vi "Choreo_Choreo_DifferentialLTVCommand.vi"(4 "Pass_Through_Time":dbl=-1.0 format="%33.4f", 5 "TimePastEndSeconds":dbl=3.0, 6 "FlipIfNeeded":bool=TRUE, 8 "Auto":bool=TRUE, 9 "Initialize":bool, 10 "TrajectoryName":string, 11 "Current Position":T3={"TRANSLATION"={"X"=0.0, "Y"=0.0}, "ROTATION"={"VALUE"=0.0, "COS"=1.0, "SIN"=0.0}} {"ROTATION"."SIN" format="%13.4f"; "ROTATION"."COS" format="%13.4f"; "ROTATION"."VALUE" format="%13.4f"; "TRANSLATION"."Y" format="%14.3f"; "TRANSLATION"."X" format="%14.3f"}) -> (0 "Ctrl Info":T1, 1 "Complete":bool, 2 "On Target":bool, 3 "Chassis Speed Dmd":T2 {"vOmega" format="%10.3f"; "vY" format="%10.3f"; "vX" format="%10.3f"})   [LabVIEW 2019, in "ChoreoLib.lvlib"]
doc: "Command to assist in the execution of a Choreo Trajectory. This wraps the ChoreoDifferentialLTVCtrl VI.\n\nInputs:\n - TimePastEndSeconds - double - Number of seconds past the end of the trajectory to continue to control robot position. (Optional. Default: 3.0 )\n - Current Pose - pose2d - Current robot position pose calcualted by either Odometry or Pose Estimation.\n - TrajectoryName - string - Name of trajectory to load from cache. If it isn't in cache, it will try to be loaded from the file system.\n - Initialize - boolean - Set to true for one scan cycle when starting a trajectory. Resets the elapsed time and controllers.\n - Auto - boolean - When TRUE closed loop control is used to control trajectory execution. This is mostly for debugging and robot tuning. (Optional. Default: TRUE )\n - Mirror For Red Alliance - boolean - Whether or not to mirror the path based on alliance (this assumes the path is created for the blue alliance) If TRUE, the alliance color is queried and if RED, the trajectory is flipped for execution.\n - PassThroughTime - double - Continueually counting time (seconds) read from the FGPA on roboRIO or local computer when running on PC. (Optional: Default: Read FGPA time )\n\nOutputs:\n - Choreo Speed Demand - chassis speed - Desired chassis speed (M/S, Rad/Sec)\n - On Target - boolean - TRUE when robot position is within tolerance of trajectory position\n - Complete - boolean - TRUE when trajectory time has elapsed and robot is on target or when trajectory time is \"TimePastEndSeconds\" past trajectory end time regardless of On Target status.\n - Ctrl Info - cluster - Information on control. Mostly for diagnostics."
uses:
  ChoreoLib.lvlib
  <vilib>/Rock Robotics/WPI/ThirdParty/JAS_Junk/TrajLib/TypeDef/POSE2D.ctl
  <vilib>/Rock Robotics/WPI/ThirdParty/JAS_Junk/TrajLib/TypeDef/TRANSLATION2D.ctl
  <vilib>/Rock Robotics/WPI/ThirdParty/JAS_Junk/TrajLib/TypeDef/ROTATION2D.ctl
  <vilib>/Rock Robotics/WPI/ThirdParty/JAS_Junk/TrajLib/TypeDef/CHASSIS_SPEEDS.ctl
  TypeDef/ChoreoTrajectoryDifferential.ctl
  TypeDef/ChoreoDifferentialSample.ctl
  TypeDef/ChoreoEventMarker.ctl
  <vilib>/Rock Robotics/WPI/ThirdParty/JAS_Junk/TrajLib/VI/Util_GetTime_U32.vi
  Choreo_TrajectoryDifferential_Samples.vi
  Choreo_DifferentialSample_GetTimestamp.vi
  <vilib>/Rock Robotics/WPI/ThirdParty/JAS_Junk/TrajLib/VI/Util_GetTime_U64.vi
  <vilib>/Rock Robotics/WPI/DriverStation/WPI_DriverStationGet Alliance Info.vi
  <vilib>/Rock Robotics/WPI/ThirdParty/JAS_Junk/TrajLib/Trajectory_Library.lvlib
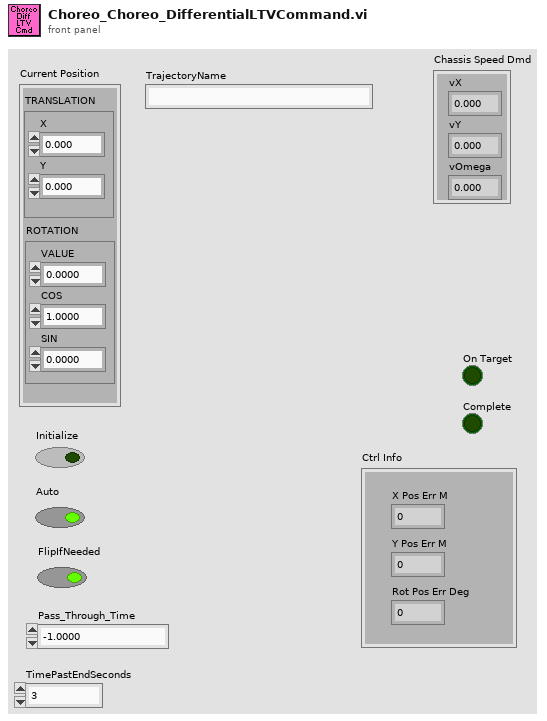
[diagram p1: front panel]
types:
  T1 = cluster{"X Pos Err M":dbl, "Y Pos Err M":dbl, "Rot Pos Err Deg":dbl}
  T2 = typedef "Trajectory_Library.lvlib/CHASSIS_SPEEDS.ctl" = cluster{"vX":dbl, "vY":dbl, "vOmega":dbl}
  T3 = typedef "Trajectory_Library.lvlib/POSE2D.ctl" = cluster{"TRANSLATION":T4, "ROTATION":T5}
  T4 = typedef "Trajectory_Library.lvlib/TRANSLATION2D.ctl" = cluster{"X":dbl, "Y":dbl}
  T5 = typedef "Trajectory_Library.lvlib/ROTATION2D.ctl" = cluster{"VALUE":dbl, "COS":dbl, "SIN":dbl}
  T6 = typedef "ChoreoLib.lvlib/ChoreoTrajectoryDifferential.ctl" = cluster{"name":string, "samples":T7[], "splits":i32[], "events":T8[]}
  T7 = typedef "ChoreoLib.lvlib/ChoreoDifferentialSample.ctl" = cluster{"timestamp":dbl, "x":dbl, "y":dbl, "heading":dbl, "velocityL":dbl, "velocityR":dbl, "angularVelocity":dbl, "accelL":dbl, "accelR":dbl, "accelAngular":dbl, "forceL":dbl, "forceR":dbl}
  T8 = typedef "ChoreoLib.lvlib/ChoreoEventMarker.ctl" = cluster{"TimeStamp":dbl, "Name":string}
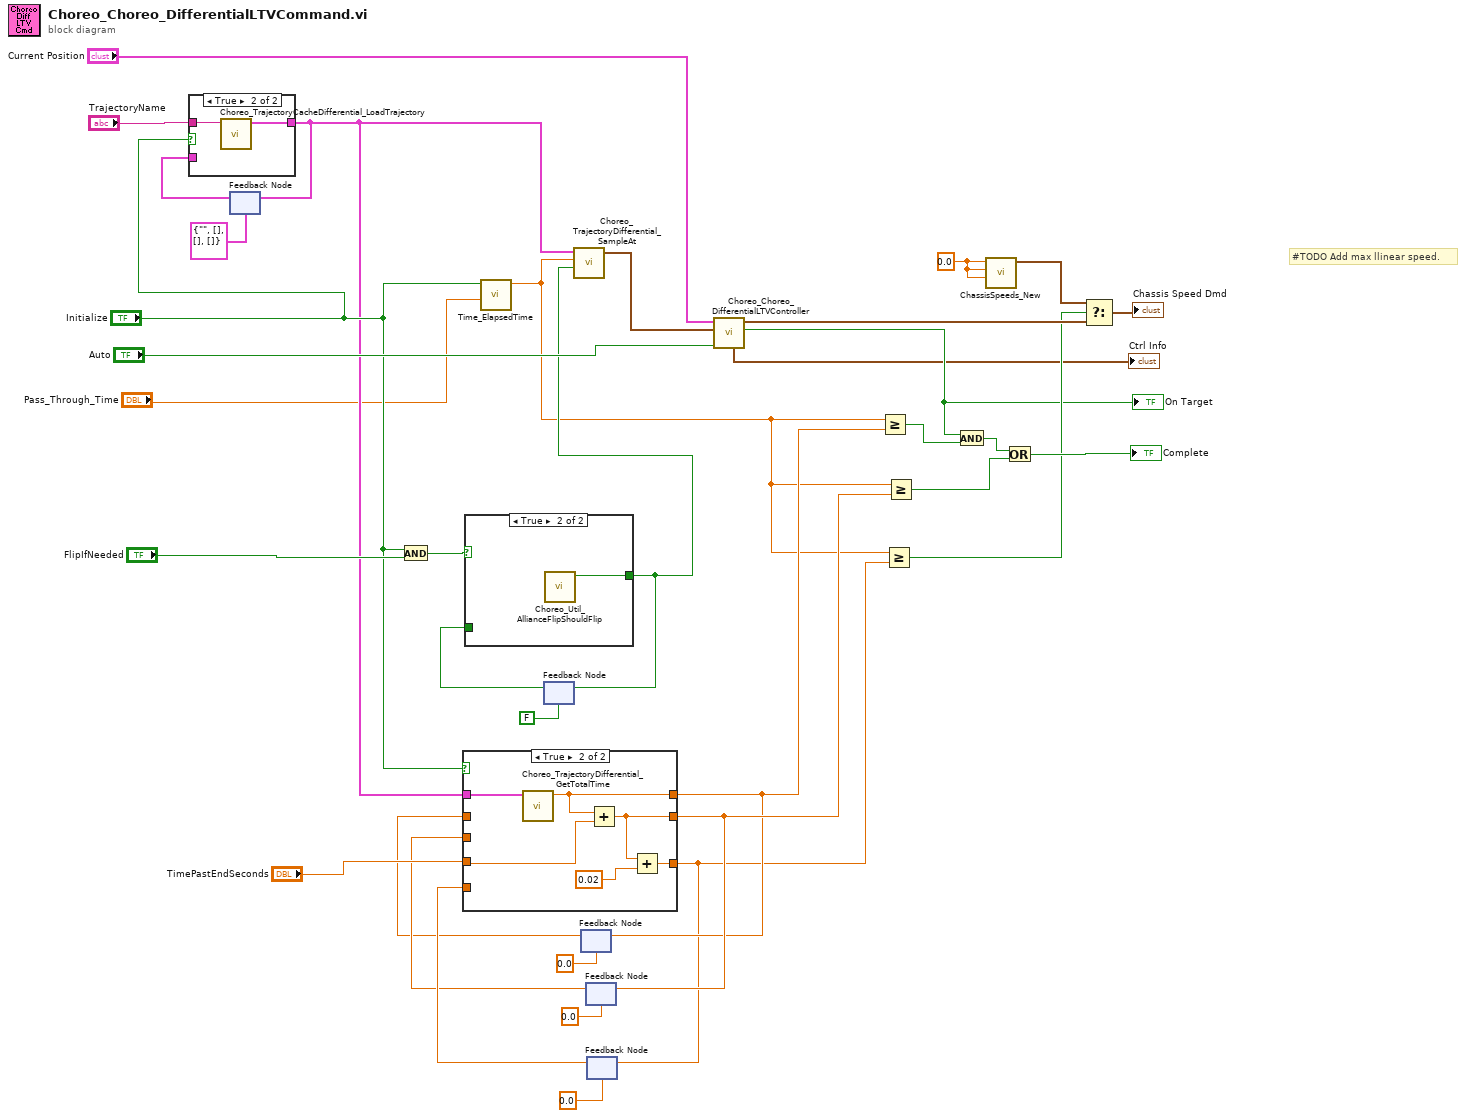
[diagram p0: block diagram]
diagram:
  w10 = 0.0 ("vX")
  # "#TODO Add max llinear speed."
  n1 = feedback #1(T6 {"name"="", "samples"=[], "splits"=[], "events"=[]} ("ChoreoTrajectoryDifferential")) -> (w4:T6)
  n2 = case shown="True" "Initialize" {
    tunnel: [w37 w39] -> w5
    tunnel: "TrajectoryName" -> [_ w38]
    tunnel: w4 -> [w37 _]
    frame False {
    }
    frame True {
      n3 = call "Choreo_TrajectoryCacheDifferential_LoadTrajectory.vi"("TrajectoryName"=w38) -> ("ChoreoTrajectoryDifferential"=w39:T6)  [unwired: 9 in, 1 out]
    }
  }
  n4 = feedback-in #1(w5) -> ()
  n5 = And(x="Initialize", y="FlipIfNeeded") -> (x .and. y?=w32:bool)
  n6 = call <vilib>:"Time_ElapsedTime.vi"("PassthroughTime_SEC"="Pass_Through_Time", "Reset"="Initialize") -> ("Elapsed Time Sec"=w16:dbl)  [unwired: 9 in]
  n7 = feedback #2(FALSE) -> (w30:bool)
  n8 = case shown="True" w32 {
    tunnel: [w40 w41] -> w29
    tunnel: w30 -> [w40 _]
    frame False {
    }
    frame True {
      n9 = call "Choreo_Util_AllianceFlipShouldFlip.vi"() -> ("ShouldFlip"=w41:bool)  [unwired: 11 in]
    }
  }
  n10 = feedback-in #2(w29) -> ()
  n11 = call "Choreo_TrajectoryDifferential_SampleAt.vi"("MirrorForRedAlliance"=w29, "TimeStamp"=w16, "ChoreoTrajectoryDifferential"=w5) -> ("ChoreoDifferentialSample"=w35:T7)  [unwired: 8 in]
  n12 = feedback #3(0.0) -> (w17:dbl)
  n13 = feedback #4(0.0) -> (w24:dbl)
  n14 = feedback #5(0.0) -> (w25:dbl)
  n15 = case shown="True" "Initialize" {
    tunnel: w5 -> [_ w46]
    tunnel: "TimePastEndSeconds" -> [_ w50]
    tunnel: [w43 w49] -> w20
    tunnel: [w44 w47] -> w15
    tunnel: w25 -> [w44 _]
    tunnel: w24 -> [w43 _]
    tunnel: [w42 w45] -> w18
    tunnel: w17 -> [w42 _]
    frame False {
    }
    frame True {
      n16 = call "Choreo_TrajectoryDifferential_GetTotalTime.vi"("ChoreoTrajectoryDifferential"=w46) -> ("TotalTime"=w45:dbl)  [unwired: 10 in]
      n17 = Add(x=w45, y=w50) -> (x+y=w49:dbl)
      n18 = Add(x=w49, y=0.02) -> (x+y=w47:dbl)
    }
  }
  n19 = feedback-in #3(w18) -> ()
  n20 = feedback-in #4(w20) -> ()
  n21 = feedback-in #5(w15) -> ()
  n22 = call "Choreo_Choreo_DifferentialLTVController.vi"("Auto"="Auto", "ChoreoDifferentialSample"=w35, "Current Position"="Current Position") -> ("On Target"=w8:bool, "Chassis Speed Dmd"=w14:T2, "Ctrl Info"=→"Ctrl Info":T1)  [unwired: 6 in]
  "On Target" <- w8
  n23 = Greater Or Equal?(x=w16, y=w18) -> (x >= y?=w9:bool)
  n24 = Greater Or Equal?(x=w16, y=w15) -> (x >= y?=w13:bool)
  n25 = Greater Or Equal?(x=w16, y=w20) -> (x >= y?=w22:bool)
  n26 = And(x=w8, y=w9) -> (x .and. y?=w23:bool)
  n27 = call <vilib>:"ChassisSpeeds_New.vi"("vAngular"=w10, "vY"=w10, "vX"=w10) -> ("CHASSIS"=w11:T2)  [unwired: 8 in]
  n28 = Or(x=w23, y=w22) -> (x .or. y?=→"Complete":bool)
  n29 = Select(t=w11, s=w13, f=w14) -> (s? t:f=→"Chassis Speed Dmd":T2)
